vi "CameraXYusingGantryHeadXY.vi"(2 "GantryY":dbl, 3 "GantryX":dbl) -> (0 "CamY":dbl, 1 "CamX":dbl)   [LabVIEW 2019]
panel:
  in  "GHtoCamOffsetYmm":dbl=-11.479
  in  "GHtoCamOffsetXmm":dbl=-120.252
  # "See what is under gantry head.\nGet cocordinates using gantry head position to camera position"
  # "Constants here"
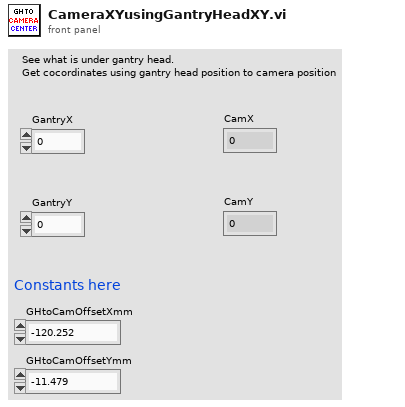
[diagram p1: front panel]
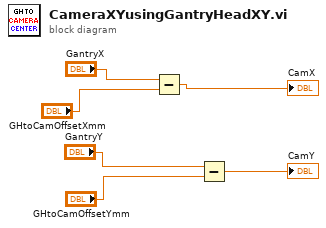
[diagram p0: block diagram]
diagram:
  n1 = Subtract(x="GantryX", y="GHtoCamOffsetXmm") -> (x-y=→"CamX":dbl)
  n2 = Subtract(x="GantryY", y="GHtoCamOffsetYmm") -> (x-y=→"CamY":dbl)
